vi "GCode Parser.vi"(8 "error in (no error)":errorcluster, 9 "Comment char":string[](array[string])=[";", "("], 10 "Search Tokens":string[](array[string])=["G", "M", "X", "Y", "Z", "I", "J", "S", "F", "E", "N"], 11 "String in":string) -> (0 "error out":errorcluster, 1 "String Array":string[](array[string]), 3 "Command Array":T1[](array[typedef]))   [LabVIEW 2014]
doc: "This GCode parser extracts the GCode commands into an \"Command Array\". Command Array contains the parameters for each command."
uses:
  GCode Command Cluster.ctl
panel:
  # "USE EOL as end."
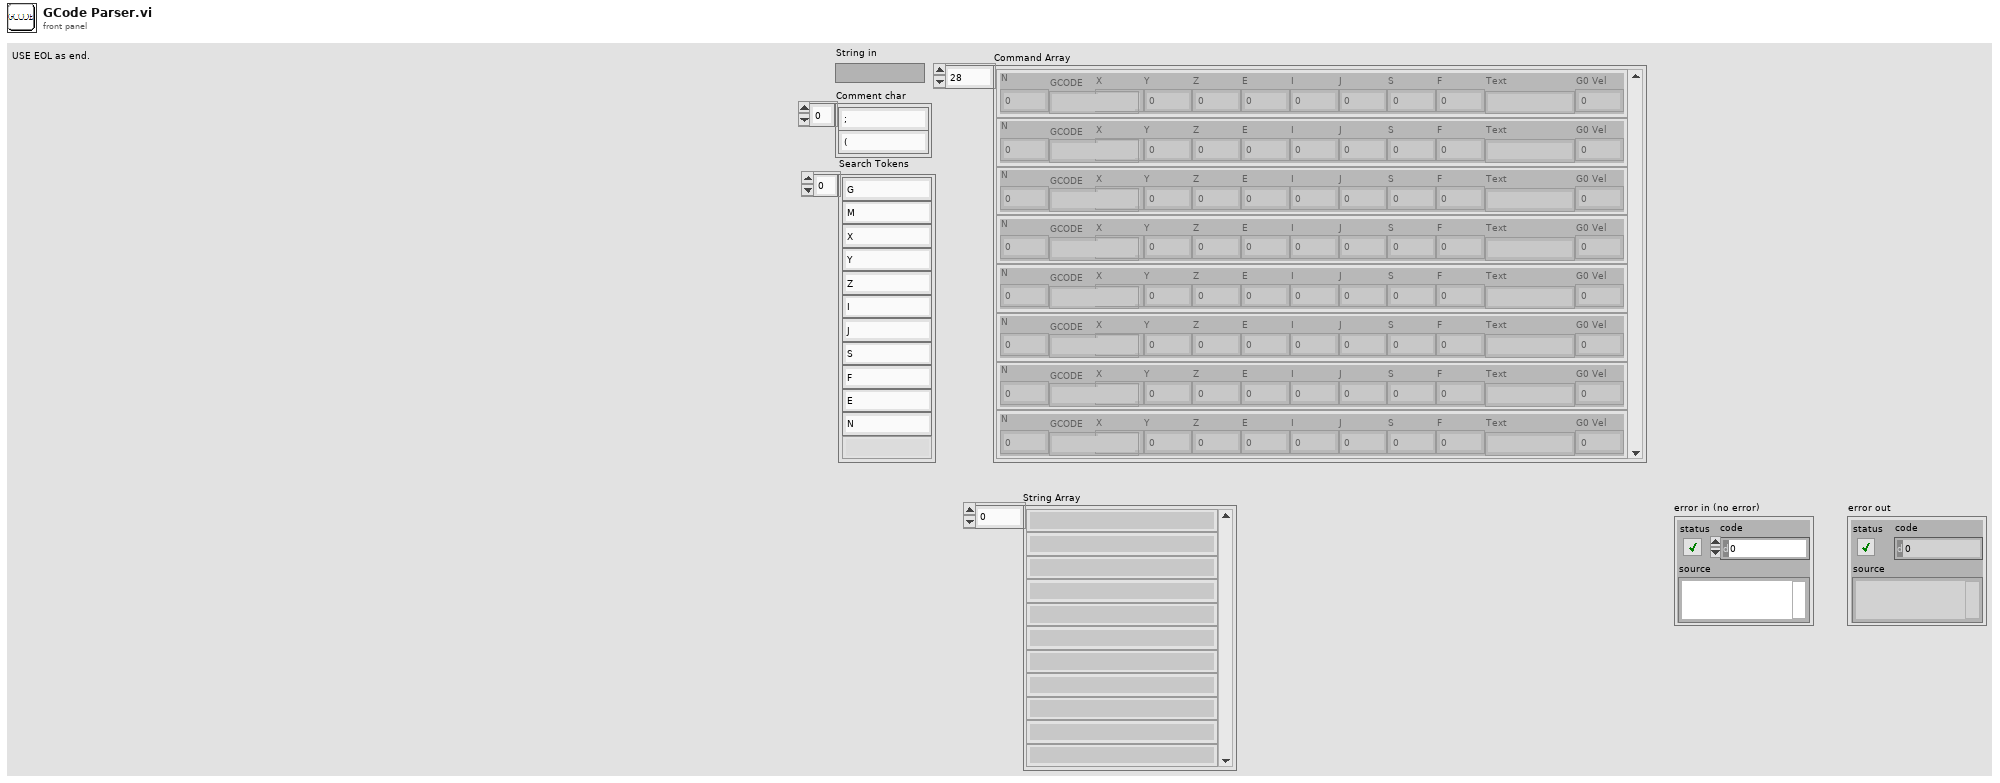
[diagram p1: front panel]
types:
  T1 = typedef "GCode Command Cluster.ctl" = cluster{"N":dbl, "GCODE":string, "X":dbl, "Y":dbl, "Z":dbl, "E":dbl, "I":dbl, "J":dbl, "S":dbl, "F":dbl, "Text":string, "G0 Vel":dbl}
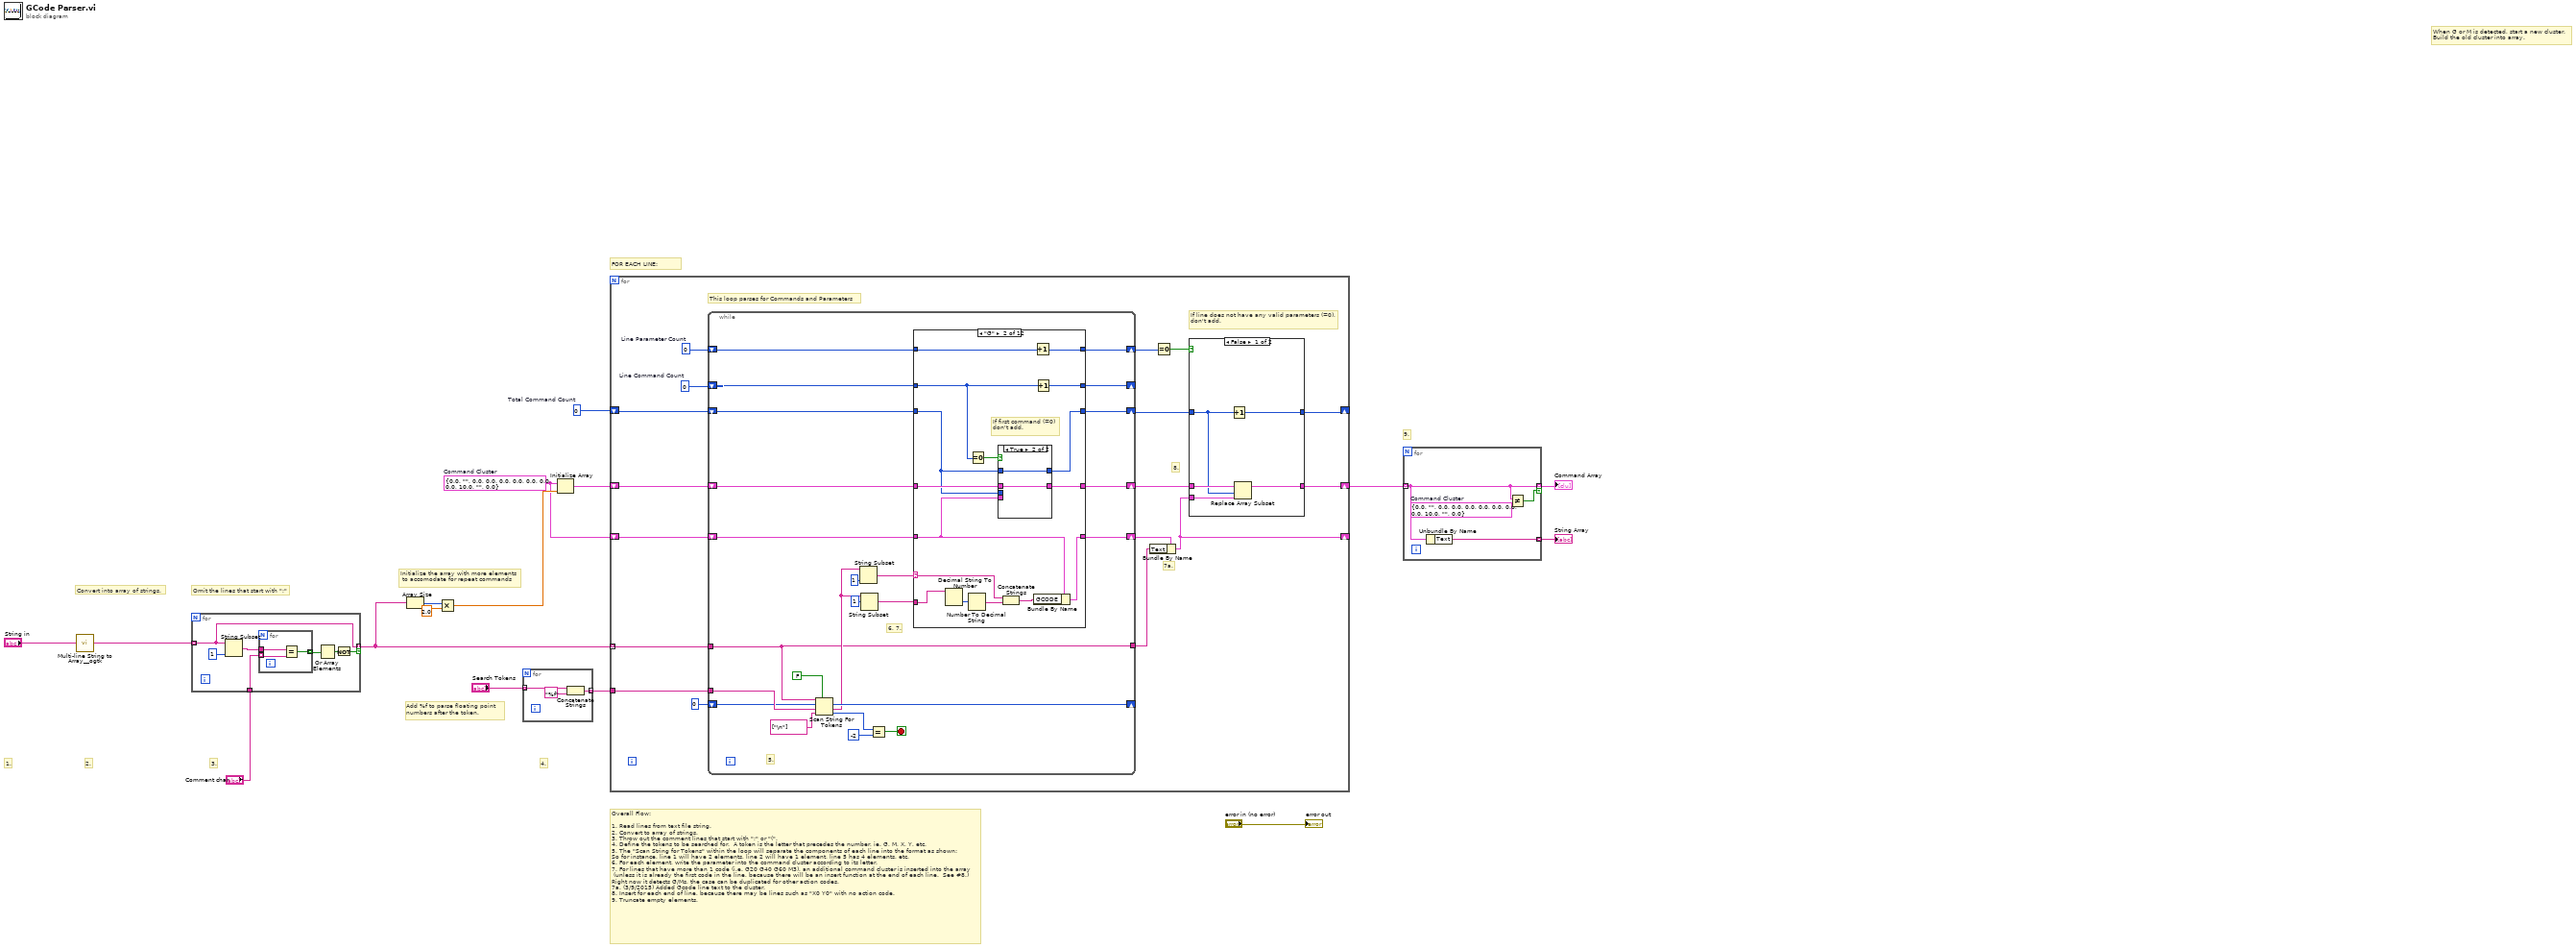
[diagram p0: block diagram]
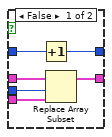
[diagram p4: hidden frame]
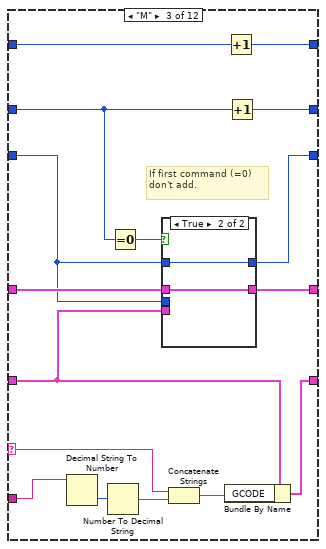
[diagram p5: hidden frame]
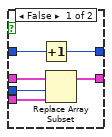
[diagram p6: hidden frame]
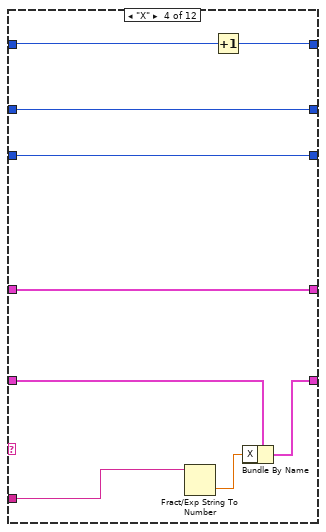
[diagram p7: hidden frame]
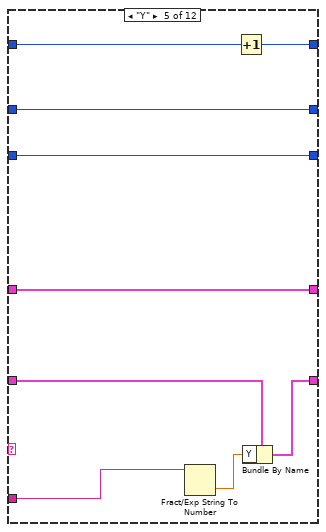
[diagram p8: hidden frame]
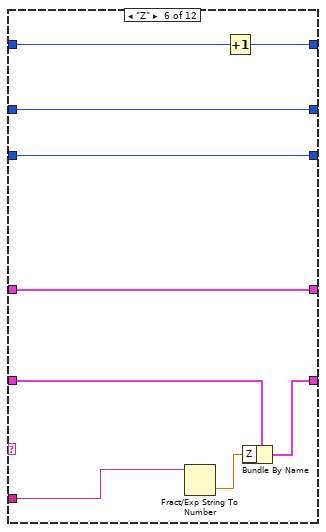
[diagram p9: hidden frame]
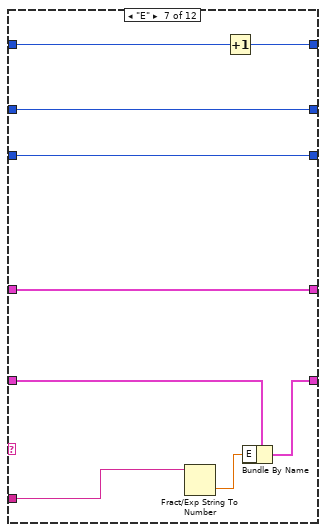
[diagram p10: hidden frame]
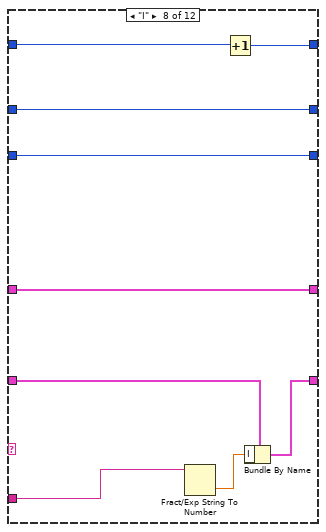
[diagram p11: hidden frame]
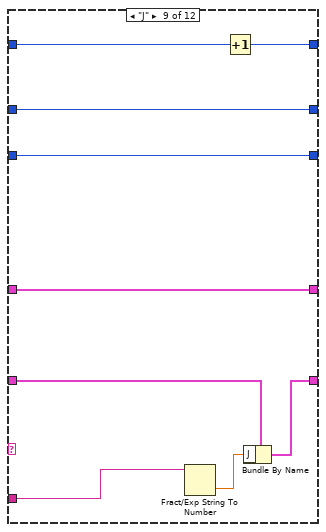
[diagram p12: hidden frame]
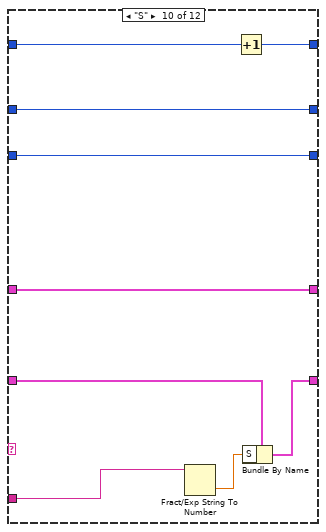
[diagram p13: hidden frame]
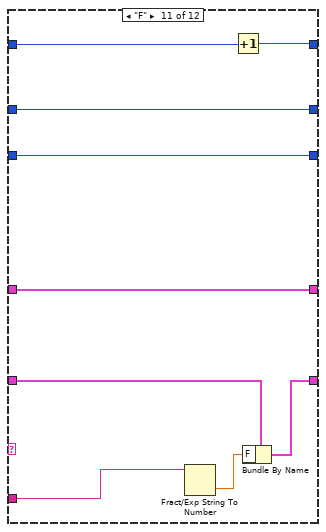
[diagram p14: hidden frame]
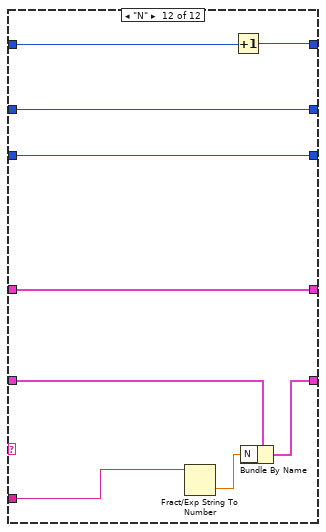
[diagram p15: hidden frame]
diagram:
  w8 = T1 {"N"=0.0, "GCODE"="", "X"=0.0, "Y"=0.0, "Z"=0.0, "E"=0.0, "I"=0.0, "J"=0.0, "S"=0.0, "F"=10.0, "Text"="", "G0 Vel"=0.0}  # Command Cluster
  w12 = 0  # Total Command Count
  # "9."
  # "Initialize the array with more elements\n to accomodate for repeat commands"
  # "Convert into array of strings."
  # "4."
  # "3."
  # "2."
  # "1."
  # "Overall Flow:\n\n1.\tRead lines from text file string.\n2.\tConvert to array of strings.\n3.\tThrow out the comment lines that start with \";\" or \"(\". \n4.\tDefine the tokens to be searched for.  A token is the letter that precedes the number, ie. G, M, X, Y, etc.\n5.\tThe \"Scan String for Tokens\" within the loop will separate the components of each line into the format as shown: \nSo for instance, line 1 will have 2 elements, line 2 will have 1 element, line 5 has 4 elements, etc.\n6.\tFor each element, write the parameter into the command cluster according to its letter.\n7.\tFor lines that have more than 1 code (i.e. G20 G40 G60 M3), an additional command cluster is inserted into the array\n (unless it is already the first code in the line, because there will be an insert function at the end of each line.  See #8.)  \nRight now it detects G/Ms, the case can be duplicated for other action codes.\n7a. (3/9/2015) Added Gcode line text to the cluster. \n8.\tInsert for each end of line, because there may be lines such as \"X0 Y0\" with no action code.\n9. Truncate empty elements."
  # "Add %f to parse floating point \nnumbers after the token."
  # "FOR EACH LINE:"
  # "Omit the lines that start with \";\""
  # "When G or M is detected, start a new cluster.\nBuild the old cluster into array."
  n1 = call "Multi-line String to Array__ogtk.vi"("string"="String in") -> ("lines"=w16:string[])
  n2 = for {
    tunnel: w16 -> [w21] mode=indexing
    tunnel: [w21] -> w2 mode=indexing if=w22
    tunnel: "Comment char" -> [w20]
    n3 = String Subset(string=w21, length (rest)=1 ("length (rest)")) -> (substring=w19:string)  [unwired: 1 in]
    n4 = for {
      tunnel: w20 -> [w25] mode=indexing
      tunnel: w19 -> [w26]
      tunnel: [w24] -> w18 mode=indexing
      n5 = Equal?(x=w26, y=w25) -> (x = y?=w24:bool)
    }
    n6 = Or Array Elements(Boolean array=w18) -> (logical OR=w17:bool)
    n7 = Not(x=w17) -> (.not. x?=w22:bool)
  }
  n8 = Array Size(array=w2) -> (size(s)=w11:i32)
  n9 = Multiply(x=w11, y=2.0) -> (x*y=w9:dbl)
  n10 = for {
    tunnel: "Search Tokens" -> [w29] mode=indexing
    tunnel: [w27] -> w14 mode=indexing
    n11 = Concatenate Strings(w29, "%f" ("string")) -> (w27:string)
  }
  n12 = Initialize Array "Initialize Array"(w8, w9) -> (w13:T1[])
  n13 = for {
    tunnel: w2 -> [w45] mode=indexing
    shift-right: [w30] -> _
    shift-left: w8 -> [w44]
    tunnel: w14 -> [w43]
    shift-right: [w33] -> w7
    shift-left: w13 -> [w42]
    shift-right: [w37] -> _
    shift-left: w12 -> [w40]
    w35 = 0  # Line Parameter Count
    w41 = 0  # Line Command Count
    # "7a."
    # "8."
    # "If line does not have any valid parameters (=0),\ndon't add."
    # "This loop parses for Commands and Parameters"
    n14 = while {
      tunnel: w43 -> [w77]
      tunnel: w45 -> [w54]
      shift-right: [w75] -> _
      shift-left: 0 ("offset past token") -> [w76]
      shift-right: [w68] -> w32
      shift-left: w44 -> [w62]
      shift-right: [w63] -> w39
      shift-left: w42 -> [w59]
      shift-right: [w64] -> _
      shift-left: w41 -> [w65]
      shift-right: [w61] -> w38
      shift-left: w40 -> [w60]
      shift-right: [w56] -> w34
      shift-left: w35 -> [w57]
      tunnel: [w54] -> w31
      stop <- w67 stop-if-true
      # "6, 7."
      # "5."
      n15 = Scan String For Tokens(5:FALSE ("allow empty tokens? (F)"), 6:string[] ["\n"] ("delimiters (\\s,\\t,\\r,\\n)"), 7:w77, 8:w76, 9:w54) -> (0:w73:i32, 1:w55:string, 2:w75:i32)  [unwired: 1 in, 1 out]
      n16 = String Subset(string=w55, length (rest)=1 ("length (rest)")) -> (substring=w70:string)  [unwired: 1 in]
      n17 = String Subset(string=w55, offset (0)=1) -> (substring=w69:string)  [unwired: 1 in]
      n18 = Equal?(x=w73, y=-2) -> (x = y?=w67:bool)
      n19 = case shown="\"G\"" w70 {
        selector: w70 -> [_ w84 w108 _ _ _ _ _ _ _ _ _]
        tunnel: [w82 w98 w122 w139 w148 w157 w166 w175 w184 w193 w202 w211] -> w68
        tunnel: w69 -> [_ w87 w107 w137 w146 w155 w164 w173 w182 w191 w200 w209]
        tunnel: w62 -> [w82 w94 w118 w136 w145 w154 w163 w172 w181 w190 w199 w208]
        tunnel: w65 -> [w81 w95 w119 w135 w144 w153 w162 w171 w180 w189 w198 w207]
        tunnel: [w81 w93 w117 w135 w144 w153 w162 w171 w180 w189 w198 w207] -> w64
        tunnel: w59 -> [w80 w96 w120 w134 w143 w152 w161 w170 w179 w188 w197 w206]
        tunnel: [w80 w97 w121 w134 w143 w152 w161 w170 w179 w188 w197 w206] -> w63
        tunnel: w60 -> [w79 w92 w116 w133 w142 w151 w160 w169 w178 w187 w196 w205]
        tunnel: [w79 w91 w115 w133 w142 w151 w160 w169 w178 w187 w196 w205] -> w61
        tunnel: w57 -> [w78 w89 w113 w132 w141 w150 w159 w168 w177 w186 w195 w204]
        tunnel: [w78 w88 w112 w131 w140 w149 w158 w167 w176 w185 w194 w203] -> w56
        frame Default {
        }
        frame "G" {
          # "If first command (=0)\ndon't add."
          n20 = Decimal String To Number(string=w87) -> (number=w86:i32)  [unwired: 2 in, 1 out]
          n21 = Number To Decimal String(number=w86) -> (decimal integer string=w85:string)  [unwired: 1 in]
          n22 = Equal To 0?(x=w95) -> (x = 0?=w90:bool)
          n23 = case shown="True" w90 {
            tunnel: w94 -> [w104 _]
            tunnel: [w102 w106] -> w97
            tunnel: w96 -> [w103 w106]
            tunnel: w92 -> [w101 _]
            tunnel: w92 -> [w100 w105]
            tunnel: [w99 w105] -> w91
            frame False {
              n24 = Increment(x=w100) -> (x+1=w99:i32)
              n25 = Replace Array Subset(array=w103, new element=w104, index=w101) -> (w102:T1[])
            }
            frame True {
            }
          }
          n26 = Concatenate Strings(w84, w85) -> (w83:string)
          n27 = Bundle By Name(cluster=w94, "GCODE"=w83) -> (w98:T1)
          n28 = Increment(x=w89) -> (x+1=w88:i32)
          n29 = Increment(x=w95) -> (x+1=w93:i32)
        }
        frame "M" {
          # "If first command (=0)\ndon't add."
          n30 = Decimal String To Number(string=w107) -> (number=w111:i32)  [unwired: 2 in, 1 out]
          n31 = Number To Decimal String(number=w111) -> (decimal integer string=w110:string)  [unwired: 1 in]
          n32 = Equal To 0?(x=w119) -> (x = 0?=w114:bool)
          n33 = case shown="True" w114 {
            tunnel: w118 -> [w128 _]
            tunnel: [w126 w130] -> w121
            tunnel: w120 -> [w127 w130]
            tunnel: w116 -> [w125 _]
            tunnel: w116 -> [w124 w129]
            tunnel: [w123 w129] -> w115
            frame False {
              n34 = Increment(x=w124) -> (x+1=w123:i32)
              n35 = Replace Array Subset(array=w127, new element=w128, index=w125) -> (w126:T1[])
            }
            frame True {
            }
          }
          n36 = Concatenate Strings(w108, w110) -> (w109:string)
          n37 = Bundle By Name(cluster=w118, "GCODE"=w109) -> (w122:T1)
          n38 = Increment(x=w113) -> (x+1=w112:i32)
          n39 = Increment(x=w119) -> (x+1=w117:i32)
        }
        frame "X" {
          n40 = Fract/Exp String To Number(string=w137) -> (number=w138:dbl)  [unwired: 3 in, 1 out]
          n41 = Increment(x=w132) -> (x+1=w131:i32)
          n42 = Bundle By Name(cluster=w136, "X"=w138) -> (w139:T1)
        }
        frame "Y" {
          n43 = Fract/Exp String To Number(string=w146) -> (number=w147:dbl)  [unwired: 3 in, 1 out]
          n44 = Increment(x=w141) -> (x+1=w140:i32)
          n45 = Bundle By Name(cluster=w145, "Y"=w147) -> (w148:T1)
        }
        frame "Z" {
          n46 = Fract/Exp String To Number(string=w155) -> (number=w156:dbl)  [unwired: 3 in, 1 out]
          n47 = Increment(x=w150) -> (x+1=w149:i32)
          n48 = Bundle By Name(cluster=w154, "Z"=w156) -> (w157:T1)
        }
        frame "E" {
          n49 = Fract/Exp String To Number(string=w164) -> (number=w165:dbl)  [unwired: 3 in, 1 out]
          n50 = Increment(x=w159) -> (x+1=w158:i32)
          n51 = Bundle By Name(cluster=w163, "E"=w165) -> (w166:T1)
        }
        frame "I" {
          n52 = Fract/Exp String To Number(string=w173) -> (number=w174:dbl)  [unwired: 3 in, 1 out]
          n53 = Increment(x=w168) -> (x+1=w167:i32)
          n54 = Bundle By Name(cluster=w172, "I"=w174) -> (w175:T1)
        }
        frame "J" {
          n55 = Fract/Exp String To Number(string=w182) -> (number=w183:dbl)  [unwired: 3 in, 1 out]
          n56 = Increment(x=w177) -> (x+1=w176:i32)
          n57 = Bundle By Name(cluster=w181, "J"=w183) -> (w184:T1)
        }
        frame "S" {
          n58 = Fract/Exp String To Number(string=w191) -> (number=w192:dbl)  [unwired: 3 in, 1 out]
          n59 = Increment(x=w186) -> (x+1=w185:i32)
          n60 = Bundle By Name(cluster=w190, "S"=w192) -> (w193:T1)
        }
        frame "F" {
          n61 = Fract/Exp String To Number(string=w200) -> (number=w201:dbl)  [unwired: 3 in, 1 out]
          n62 = Increment(x=w195) -> (x+1=w194:i32)
          n63 = Bundle By Name(cluster=w199, "F"=w201) -> (w202:T1)
        }
        frame "N" {
          n64 = Fract/Exp String To Number(string=w209) -> (number=w210:dbl)  [unwired: 3 in, 1 out]
          n65 = Increment(x=w204) -> (x+1=w203:i32)
          n66 = Bundle By Name(cluster=w208, "N"=w210) -> (w211:T1)
        }
      }
    }
    n67 = Bundle By Name(cluster=w32, "Text"=w31) -> (w30:T1)
    n68 = Equal To 0?(x=w34) -> (x = 0?=w36:bool)
    n69 = case shown="False" w36 {
      tunnel: w39 -> [w51 w52]
      tunnel: w30 -> [w50 _]
      tunnel: [w49 w53] -> w37
      tunnel: w38 -> [w48 w53]
      tunnel: [w47 w52] -> w33
      frame False {
        n70 = Increment(x=w48) -> (x+1=w49:i32)
        n71 = Replace Array Subset "Replace Array Subset"(array=w51, new element=w50, index=w48) -> (w47:T1[])
      }
      frame True {
      }
    }
  }
  n72 = for {
    tunnel: w7 -> [w213] mode=indexing
    tunnel: [w213] -> w6 mode=indexing if=w214
    tunnel: [w212] -> w1 mode=indexing
    w215 = T1 {"N"=0.0, "GCODE"="", "X"=0.0, "Y"=0.0, "Z"=0.0, "E"=0.0, "I"=0.0, "J"=0.0, "S"=0.0, "F"=10.0, "Text"="", "G0 Vel"=0.0}  # Command Cluster
    n73 = Unbundle By Name(w213) -> ("Text"=w212:string)
    n74 = Not Equal?(x=w213, y=w215) -> (x != y?=w214:bool)
  }
  "Command Array" <- w6
  "String Array" <- w1
  "error out" <- "error in (no error)"
